vi "Do Calibration.vi"(5 "PAS Data":refnum<k24>, 7 "PasDataByGas":refnum<k24>[](array[refnum]), 8 "error in (no error)":errorcluster, 9 "pasValuesByFilter":refnum<k24>[](array[refnum]), 10 "pasDataByGas":refnum<k24>, 11 "gasID":i32) -> (0 "error out":errorcluster, 3 "calResult":refnum<k24>)   [LabVIEW 2015]
uses:
  C:/Distributed/CalFlex.dll
  CalFlex.dll
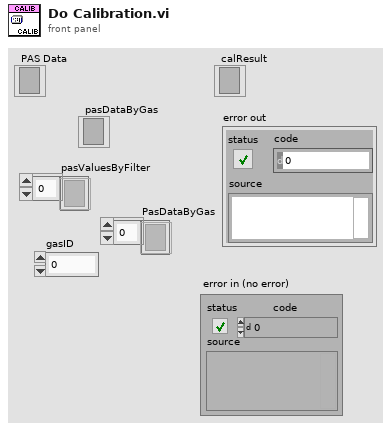
[diagram p1: front panel]
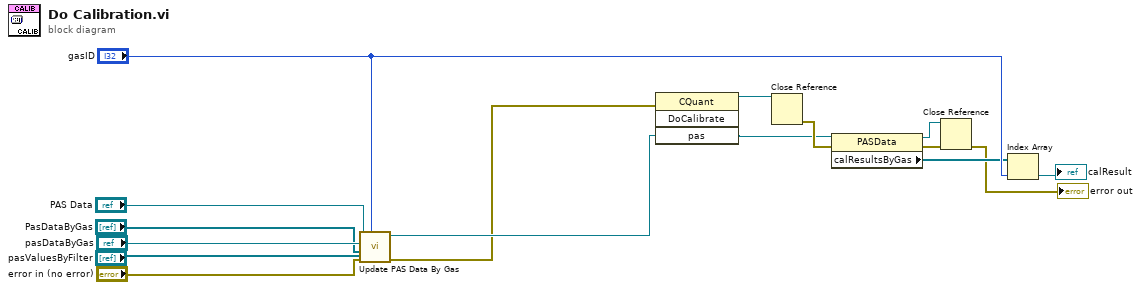
[diagram p0: block diagram]
diagram:
  n1 = call "Update PAS Data By Gas.vi"("pasValuesByFilter"="pasValuesByFilter", "gasID"="gasID", "error in (no error)"="error in (no error)", "PasDataByGas"="PasDataByGas", "pasDataByGas"="pasDataByGas", "PASData In"="PAS Data") -> ("error out"=w1:errorcluster, "PAS Data Out"=w5:refnum<k24>)  [unwired: 4 in]
  n2 = invoke class="CQuant" method="DoCalibrate"(error in=w1, "pas"=w5) -> (reference out=w4:refnum<k24>, "pas"=w3:refnum<k24>)  [unwired: 2 in, 2 out]
  n3 = Close Reference(reference=w4) -> (error out=w14:errorcluster)  [unwired: 1 in]
  n4 = property class="PASData"(reference=w3, error in=w14) -> (reference out=w11:refnum<k24>, error out=w13:errorcluster, "calResultsByGas"=w15:refnum<k24>[])
  n5 = Close Reference(reference=w11, error in (no error)=w13) -> (error out=→"error out":errorcluster)
  n6 = Index Array(array=w15, index="gasID") -> (element=→"calResult":refnum<k24>)
